vi "Log Data.vi"(8 "error in (no error)":errorcluster, 11 "MFC in":refnum<class "MFC.lvclass">) -> (0 "error out":errorcluster, 3 "MFC out":refnum<class "MFC.lvclass">)   [LabVIEW 2013, in "MFC.LVLIB" / "MFC.lvclass"]
uses:
  MFC.lvclass
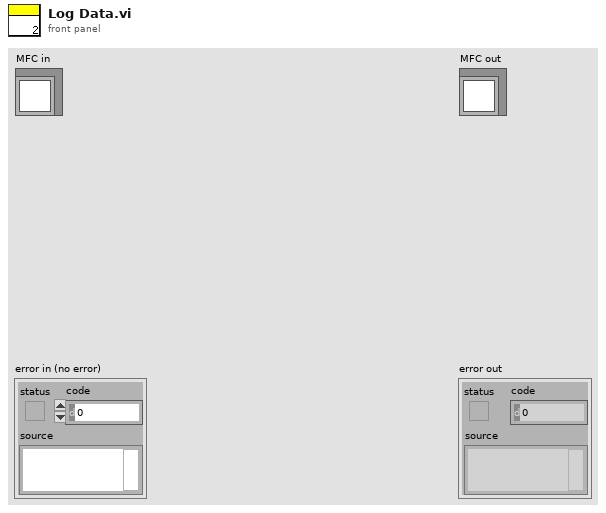
[diagram p1: front panel]
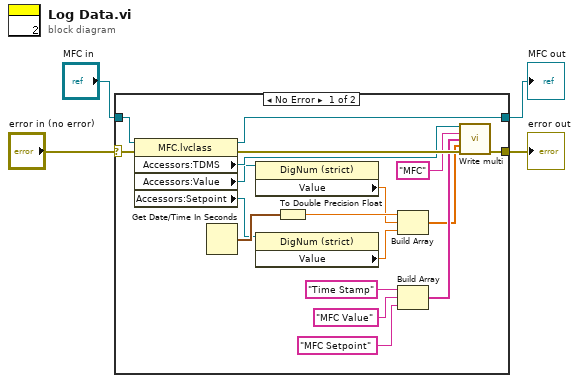
[diagram p0: block diagram]
diagram:
  n1 = case shown="No Error" "error in (no error)" {
    selector: "error in (no error)" -> [w11 w24]
    tunnel: [w10 w24] -> w3
    tunnel: [w20 w23] -> w1
    tunnel: "MFC in" -> [w21 w23]
    frame No Error {
      n2 = property class="MFC.lvclass"(reference=w21, error in=w11) -> (reference out=w20:refnum<class "MFC.lvclass">, error out=w19:errorcluster, "Accessors:TDMS"=w18:refnum<k34>, "Accessors:Value"=w9:refnum<vi>, "Accessors:Setpoint"=w8:refnum<vi>)
      n3 = Get Date/Time In Seconds() -> (seconds since 1Jan1904=w22:timestamp)
      n4 = property class="DigNum (strict)"(reference=w9) -> ("Value"=w7:dbl)  [unwired: 1 in, 2 out]
      n5 = property class="DigNum (strict)"(reference=w8) -> ("Value"=w6:dbl)  [unwired: 1 in, 2 out]
      n6 = To Double Precision Float(number=w22) -> (double precision float=w12:dbl)
      n7 = Build Array(w12, w7, w6) -> (w5:dbl[])
      n8 = Build Array("Time Stamp" ("Channel"), "MFC Value" ("string"), "MFC Setpoint" ("string")) -> (w13:string[])
      n9 = call "Write multi.vi"("tdms file in"=w18, "group"="MFC", "Channel"=w13, "Data"=w5, "error in (no error)"=w19) -> ("error out"=w10:errorcluster)  [unwired: 7 in, 3 out]
    }
    frame Error {
    }
  }
  "error out" <- w3
  "MFC out" <- w1
